vi "CLC_GEN3_L2_InPhaseCal_mW_BaseOnly.vi"() -> ()   [LabVIEW 2023, in "Clover_Cell.lvlib"]
uses:
  Clover_Cell.lvlib
  lib/Anritsu Signal Analyzer Series/Anritsu Signal Analyzer Series.lvlib
  lib/ELTA/ELTA.lvlib
panel:
  in  "Base_Gain":i32
  in  "Base_Phase":i32
  in  "Base_Ch":i32
  in  "Daul_Ch_Phase_Sweep":bool
  in  "SweepSwitch?":u16(ring) items=["NoSweep(Single)", "Sweep"]
  in  "SweepMode":u16(ring) items=["Phase", "Gain"]
  in  "Method":u16(ring)=1 items=["dBm"=1, "mW"=2]
  in  "Polarity":u16(ring) items=["H", "V"]
  in  "VISA resource name":refnum<visa-resource-name>="TCPIP0::192.168.100.230::inst0::INSTR"
  in  "CenterFreq(GHz)":dbl=28.0
  in  "AvgTimes":i32=3
  in  "Single_Ch_Phase_Sweep":bool
  in  "TRXmode":u16(ring)=1 items=["Rx"=2, "Tx"=1]
  out "GainStep":i32=63
  out "PhaseStep":i32=63
  out "Channel":i32=63
  out "Total mW":dbl format="%.7f"
  out "Total dBm":dbl format="%.7f"
  out "Ref. mW":dbl format="%.7f"
  out "Ref. dBm":dbl format="%.7f"
  out "Main mW":dbl format="%.7f"
  out "Main dBm":dbl format="%.7f"
  out "Data":dbl[][](array[numeric])
  out "FileNAME_Single":string
  out "Spectrum Analyzer":dbl[](graph)
  out "CurrentData":dbl[](array[numeric])
  out "Duration":dbl
  out "TotalTime":dbl format="%.2f"
  out "StopTime":timestamp=timestamp(3663835912.033212 s since 1904-01-01)
  out "FileNAME_Dual":string
  out "StartTime":timestamp=timestamp(3663835741.875155 s since 1904-01-01)
  out "TX/RX":u16=1
  out "error out":errorcluster
  out "output cluster":T1={"address"="192.168.100.111", "remote port or service name"=5025, "timeout ms (60000)"=10000}
  out "Operating \nChannel(s)":bool[][](array[boolean])
  out "OK?":bool
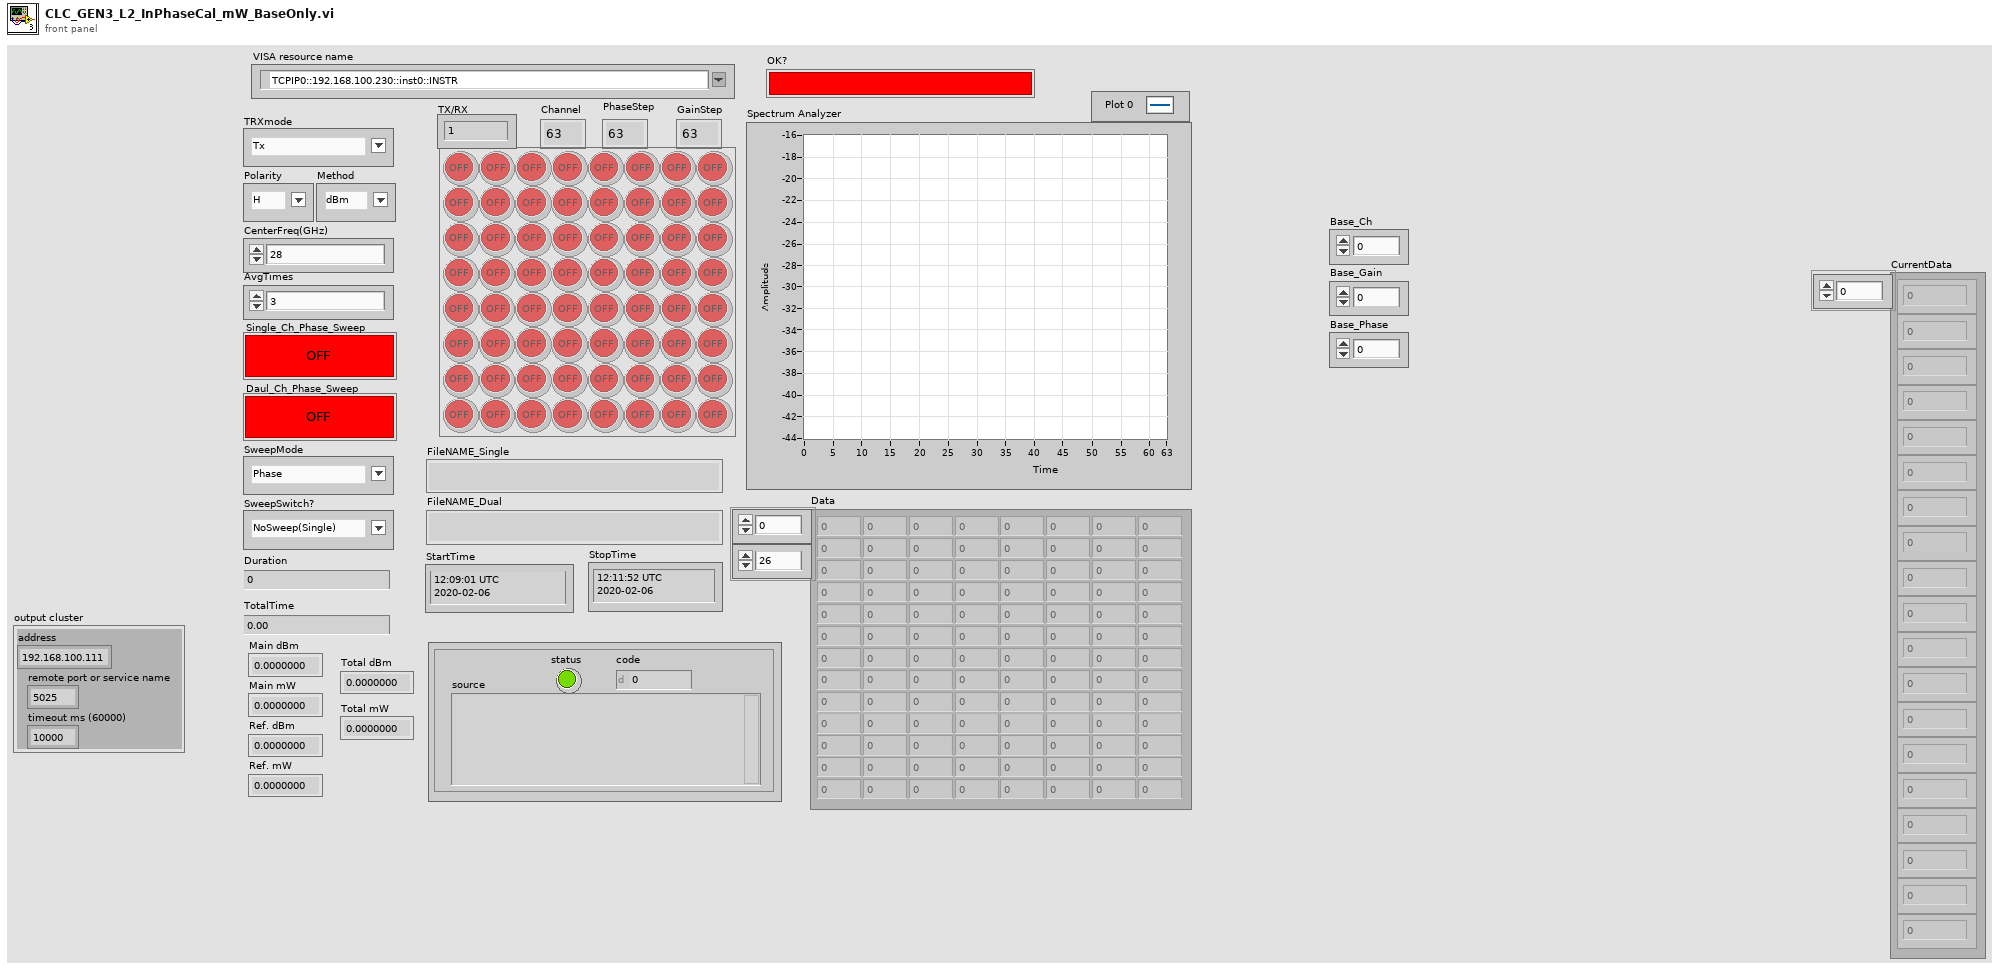
[diagram p1: front panel]
types:
  T1 = cluster{"address":string, "remote port or service name":u16, "timeout ms (60000)":i32}
  T2 = cluster{"Mode":u16, "Polarity":u16, "CH_ON/OFF":u16, "Channel":i32, "Gain":i32, "Phase":i32}
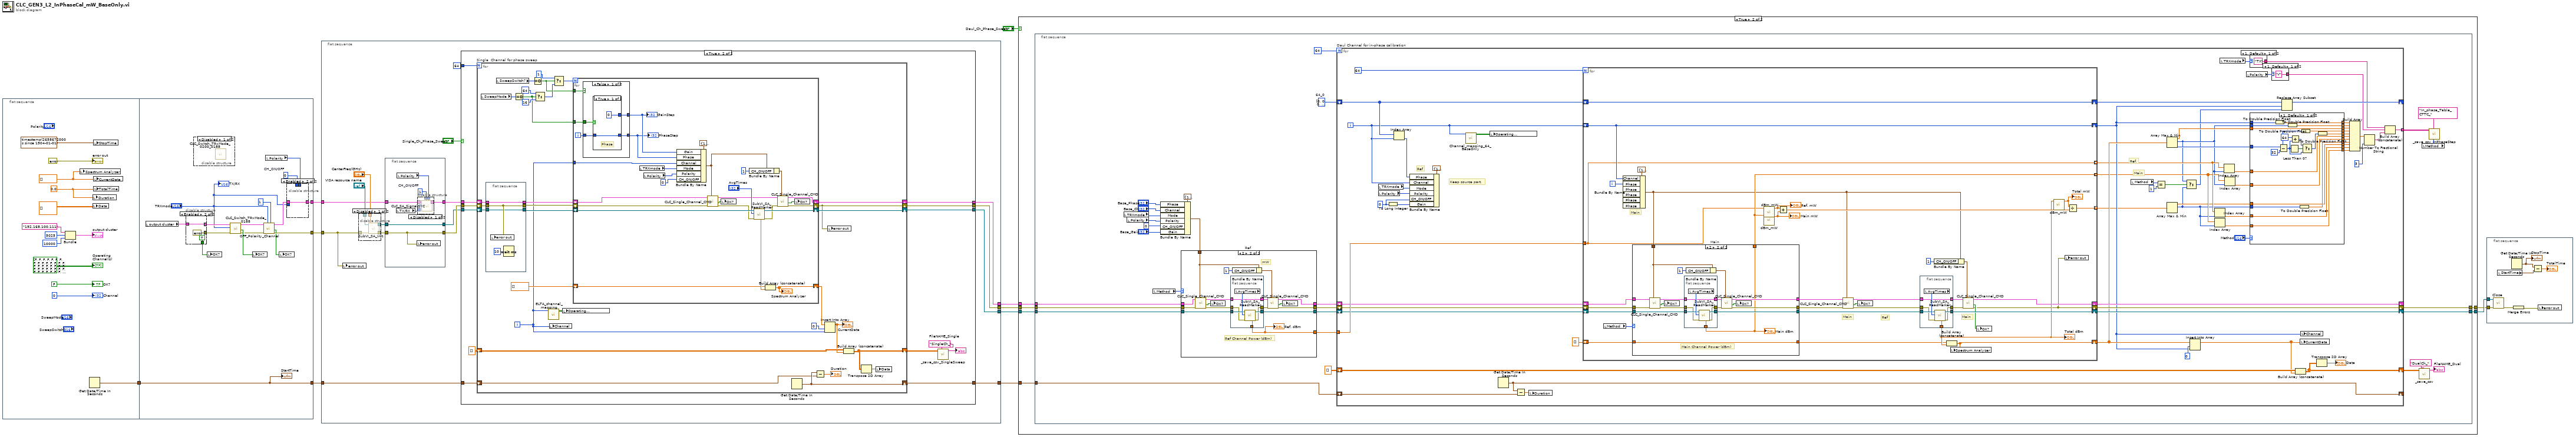
[diagram p0: block diagram]
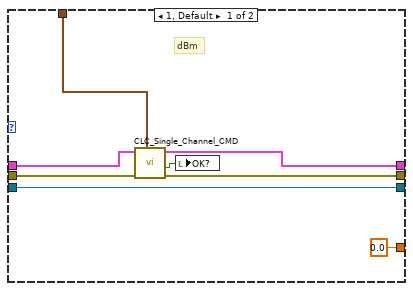
[diagram p3: hidden frame]
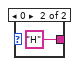
[diagram p4: hidden frame]
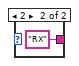
[diagram p5: hidden frame]
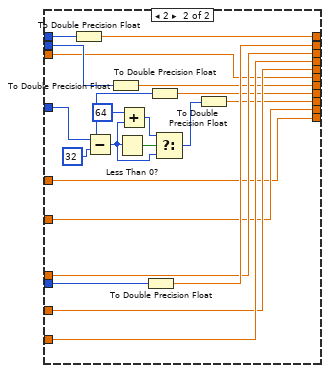
[diagram p6: hidden frame]
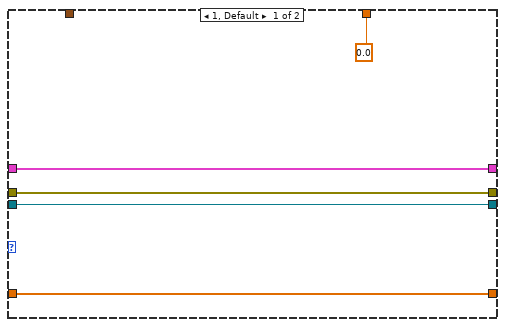
[diagram p7: hidden frame]
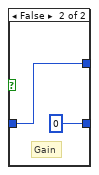
[diagram p10: hidden frame]
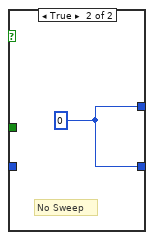
[diagram p11: hidden frame]
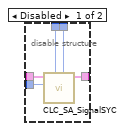
[diagram p14: hidden frame]
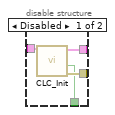
[diagram p15: hidden frame]
diagram:
  n1 = flat-sequence {
    tunnel: [w12] -> w11
    tunnel: w11 -> [w28]
    tunnel: [w31] -> w2
    tunnel: [w35] -> w3
    tunnel: [w28] -> w10
    frame #0 {
      w16 = dbl[] []
      w19 = 0.0 ("TotalTime")
      n2 = Bundle("address"="192.168.100.111", "remote port or service name"=u16 5025, "timeout ms (60000)"=10000) -> (→"output cluster":T1)  [unwired: 1 in]
      n3 = local write "Spectrum Analyzer"(w16) -> ()
      n4 = Get Date/Time In Seconds() -> (seconds since 1Jan1904=w12:timestamp)
      n5 = local write "Duration"(w19) -> ()
      n6 = local write "Data"(dbl[][] []) -> ()
      n7 = local write "StopTime"(timestamp(2658672000.001 s since 1904-01-01) ("StopTime")) -> ()
      n8 = local write "CurrentData"(w16) -> ()
      n9 = local write "TotalTime"(w19) -> ()
      "error out" <- errorcluster {"status"=FALSE, "code"=0, "source"=""} ("error out")
      "Operating \nChannel(s)" <- bool[][] [[FALSE, FALSE, FALSE, FALSE, FALSE, FALSE, FALSE, FALSE], [FALSE, FALSE, FALSE, FALSE, FALSE, FALSE, FALSE, FALSE], [FALSE, FALSE, FALSE, FALSE, FALSE, FALSE, FALSE, FALSE], [FALSE, FALSE, FALSE, FALSE, FALSE, FALSE, FALSE, FALSE], [FALSE, FALSE, FALSE, FALSE, FALSE, FALSE, FALSE, FALSE], [FALSE, FALSE, FALSE, FALSE, FALSE, FALSE, FALSE, FALSE], [FALSE, FALSE, FALSE, FALSE, FALSE, FALSE, FALSE, FALSE], [FALSE, FALSE, FALSE, FALSE, FALSE, FALSE, FALSE, FALSE]] ("Operating \nChannel(s)")
      "Channel" <- 0 ("Channel")
      "OK?" <- FALSE ("OK?")
    }
    frame #1 {
      w30 = u16 0  # CH_ON/OFF
      n10 = local read "output cluster"() -> (w40:T1)
      n11 = disable-structure shown="Enabled" {
        disable-tunnel: w40 -> [w50 w53]
        disable-tunnel: [w49 w53] -> w39
        disable-tunnel: [w48 errorcluster {"status"=FALSE, "code"=0, "source"=""} ("error in (no error)")] -> w37
        disable-tunnel: [w47 TRUE ("OK?")] -> w29
        frame Disabled {
          n12 = call "CLC_Init.vi"("TCPIPin"=w50) -> ("error out"=w48:errorcluster, "Status"=w47:bool, "TCPIPin 2"=w49:T1)  [unwired: 8 in]
        }
        frame Enabled {
        }
      }
      n13 = disable-structure shown="Disabled" {
        frame Disabled {
          n14 = call "CLC_Switch_TRxMode_0200_0188.vi"() -> ()  [unwired: 9 in, 3 out]
        }
        frame Enabled {
        }
      }
      n15 = local write "OK?"(w29) -> ()
      n16 = call "CLC_Switch_TRxMode_0188.vi"("error in (no error)"=w37, "Text Ring"="TRXmode", "TCPIPin"=w39) -> ("error out"=w36:errorcluster, "OK?"=w38:bool, "TCPIPin 2"=w34:T1)  [unwired: 6 in]
      n17 = local write "OK?"(w38) -> ()
      n18 = call "OFF_Polarity_Channel.vi"("CH_ON:0/OFF:1"=u16 1, "Mode"="TRXmode", "error in"=w36, "TCPIPin"=w34) -> ("error out"=w35:errorcluster, "OK?"=w33:bool, "TCPIPout"=w32:T1)  [unwired: 5 in]
      n19 = local read "Polarity"() -> (w26:u16)
      n20 = local write "OK?"(w33) -> ()
      n21 = disable-structure shown="Enabled" {
        disable-tunnel: w32 -> [w45 w46]
        disable-tunnel: [w44 w46] -> w31
        disable-tunnel: w30 -> [w43 _]
        disable-tunnel: w26 -> [w42 _]
        disable-tunnel: "TRXmode" -> [w41 _]
        frame Disabled {
          n22 = call "CLC_SA_SignalSYC.vi"("Polarity"=w42, "CH_ON/OFF"=w43, "Mode"=w41, "TCPIPin"=w45) -> ("TCPIPout"=w44:T1)  [unwired: 7 in]
        }
        frame Enabled {
        }
      }
      "StartTime" <- w28
      "TX/RX" <- "TRXmode"
    }
  }
  n23 = flat-sequence {
    tunnel: w10 -> [w67]
    tunnel: [w66] -> w9
    tunnel: [w65] -> w8
    tunnel: [w64] -> w7
    tunnel: [w63] -> w4
    tunnel: w3 -> [w61]
    tunnel: w2 -> [w58]
    frame #0 {
      n24 = local write "error out"(w61) -> ()
      n25 = disable-structure shown="Disabled" {
        disable-tunnel: "VISA resource name" -> [w74 w75]
        disable-tunnel: [w73 w76] -> w62
        disable-tunnel: w61 -> [w72 w76]
        disable-tunnel: "CenterFreq(GHz)" -> [w71 _]
        disable-tunnel: [w70 w75] -> w57
        frame Disabled {
          n26 = call "SubVI_SA_Init.vi"("error in (no error)"=w72, "CenterFreq(GHz) 2"=w71, "VISA resource name"=w74) -> ("error out 2"=w73:errorcluster, "VISA resource name out"=w70:refnum<visa-resource-name>)  [unwired: 6 in, 1 out]
        }
        frame Enabled {
        }
      }
      n27 = flat-sequence {
        tunnel: w62 -> [w171]
        tunnel: [w171] -> w59
        tunnel: w58 -> [w169]
        tunnel: w57 -> [w170]
        tunnel: [w170] -> w56
        tunnel: [w168] -> w55
        frame #0 {
          w167 = u16 1  # CH_ON/OFF
          n28 = local read "TX/RX"() -> (w165:u16)
          n29 = local read "Polarity"() -> (w166:u16)
          n30 = local write "error out"(w171) -> ()
          n31 = disable-structure shown="Disabled" {
            disable-tunnel: w169 -> [w176 w177]
            disable-tunnel: [w175 w177] -> w168
            disable-tunnel: w167 -> [w174 _]
            disable-tunnel: w166 -> [w173 _]
            disable-tunnel: w165 -> [w172 _]
            frame Disabled {
              n32 = call "CLC_SA_SignalSYC.vi"("Polarity"=w173, "CH_ON/OFF"=w174, "Mode"=w172, "TCPIPin"=w176) -> ("TCPIPout"=w175:T1)  [unwired: 7 in]
            }
            frame Enabled {
            }
          }
        }
      }
      n33 = case shown="True" "Single_Ch_Phase_Sweep" {
        tunnel: 64 -> [_ w93]
        tunnel: w67 -> [w77 w92]
        tunnel: [w78 w91] -> w66
        tunnel: [w79 w90] -> w65
        tunnel: [w80 w89] -> w64
        tunnel: [w77 w88] -> w63
        tunnel: w59 -> [w79 w87]
        tunnel: w56 -> [w78 w86]
        tunnel: w55 -> [w80 w85]
        frame False {
        }
        frame True {
          n34 = for "Single  Channel for phase sweep" {
            N: w93 -> [_]
            shift-right: [w123] -> w89
            shift-left: w85 -> [w109]
            shift-right: [w118] -> w90
            shift-left: w87 -> [w111]
            shift-right: [w122] -> w91
            shift-left: w86 -> [w108]
            shift-right: [w116] -> w82
            shift-left: dbl[][] [] -> [w117]
            shift-right: [w120] -> w88
            shift-left: w92 -> [w119]
            i -> [w94]
            n35 = local read "SweepMode"() -> (w103:u16)
            n36 = flat-sequence {
              tunnel: [w125] -> w107
              tunnel: w111 -> [w126]
              tunnel: [w126] -> w110
              tunnel: w109 -> [w125]
              tunnel: w108 -> [w124]
              tunnel: [w124] -> w106
              frame #0 {
                n37 = local write "error out"(w126) -> ()
                n38 = Wait (ms)(milliseconds to wait=u32 10) -> ()  [unwired: 1 out]
              }
            }
            n39 = local read "SweepSwitch?"() -> (w102:u16)
            n40 = Equal To 0?(x=w103) -> (x = 0?=w95:bool)
            n41 = Equal To 0?(x=w102) -> (x = 0?=w96:bool)
            n42 = Select(t=64, s=w95, f=16) -> (s? t:f=w97:i32)
            n43 = call "ELTA_channel_mapping.vi"("Ch_1_ref"=w94) -> ("Operating \nChannel(s)"=w104:bool[][])  [unwired: 10 in]
            n44 = local write "Channel"(w94) -> ()
            n45 = Select(t=1, s=w96, f=w97) -> (s? t:f=w100:i32)
            n46 = local write "Operating \nChannel(s)"(w104) -> ()
            n47 = for {
              N: w100 -> [_]
              shift-right: [w137] -> w123
              shift-left: w107 -> [w147]
              shift-right: [w139] -> w118
              shift-left: w110 -> [w149]
              shift-right: [w154] -> w122
              shift-left: w106 -> [w155]
              shift-right: [w150] -> w115
              shift-left: dbl[] [] -> [w151]
              tunnel: w94 -> [w144]
              tunnel: w96 -> [w132]
              tunnel: w95 -> [w129]
              i -> [w128]
              n48 = case shown="False" w132 {
                tunnel: [w156 w164] -> w131
                tunnel: [w157 w164] -> w130
                tunnel: w129 -> [w159 _]
                tunnel: w128 -> [w158 _]
                frame False {
                  n49 = case shown="True" w159 {
                    tunnel: w158 -> [w161 w162]
                    tunnel: [w161 0] -> w157
                    tunnel: [0 w162] -> w156
                    frame True {
                      # "Phase"
                    }
                    frame False {
                      # "Gain"
                    }
                  }
                }
                frame True {
                  w164 = 0
                  # "No Sweep"
                }
              }
              "PhaseStep" <- w130
              "GainStep" <- w131
              n50 = local read "TRXmode"() -> (w143:u16)
              n51 = local read "Polarity"() -> (w142:u16)
              n52 = Bundle By Name(cluster=T2 {"Mode"=1, "Polarity"=1, "CH_ON/OFF"=1, "Channel"=0, "Gain"=0, "Phase"=0} ("Channel params"), "Gain"=w131, "Phase"=w130, "Channel"=w144, "Mode"=w143, "Polarity"=w142, "CH_ON/OFF"=u16 0) -> (w136:T2)
              n53 = call "CLC_Single_Channel_CMD.vi"("Channel params"=w136, "error in"=w149, "TCPIPin"=w147) -> ("error out"=w148:errorcluster, "OK?"=w145:bool, "TCPIPout"=w138:T1)  [unwired: 6 in]
              n54 = local write "OK?"(w145) -> ()
              n55 = Bundle By Name(cluster=w136, "CH_ON/OFF"=u16 1) -> (w134:T2)
              n56 = call "SubVI_SA_ReadMarker.vi"("error in (no error)"=w148, "AvgTimes"="AvgTimes", "VISA resource name"=w155) -> ("error out"=w140:errorcluster, "VISA resource name out"=w154:refnum<visa-resource-name>, "Marker Power"=w152:dbl)  [unwired: 5 in, 1 out]
              n57 = Build Array (concatenate)(w151, w152) -> (w150:dbl[])
              "Spectrum Analyzer" <- w150
              n58 = call "CLC_Single_Channel_CMD.vi"("Channel params"=w134, "error in"=w140, "TCPIPin"=w138) -> ("error out"=w139:errorcluster, "OK?"=w133:bool, "TCPIPout"=w137:T1)  [unwired: 6 in]
              n59 = local write "OK?"(w133) -> ()
            }
            n60 = Get Date/Time In Seconds() -> (seconds since 1Jan1904=w120:timestamp)
            n61 = Subtract(x=w120, y=w119) -> (x-y=→"Duration":dbl)
            n62 = Insert Into Array(array=w115, index=0, new element=w94) -> (w113:dbl[])
            "CurrentData" <- w113
            n63 = local write "error out"(w118) -> ()
            n64 = Build Array (concatenate)(w117, w113) -> (w116:dbl[][])
            n65 = Transpose 2D Array(2D array=w116) -> (transposed array=w105:dbl[][])
            n66 = local write "Data"(w105) -> ()
          }
          n67 = call "_save_csv_SingleSweep.vi"("delimiter (\\t)"="SingleCh_" ("delimiter (\\t)"), "Data"=w82) -> ("FileName"=→"FileNAME_Single":string)  [unwired: 9 in]
        }
      }
    }
  }
  n68 = case shown="True" "Daul_Ch_Phase_Sweep" {
    tunnel: w9 -> [w179 w185]
    tunnel: w8 -> [w178 w184]
    tunnel: w7 -> [_ w183]
    tunnel: [w179 w182] -> w6
    tunnel: [w178 w181] -> w5
    tunnel: w4 -> [_ w180]
    frame False {
    }
    frame True {
      n69 = flat-sequence {
        tunnel: w185 -> [w198]
        tunnel: w184 -> [w194]
        tunnel: w183 -> [w195]
        tunnel: [w212] -> w182
        tunnel: [w211] -> w181
        tunnel: w180 -> [w210]
        frame #0 {
          w208 = i32[] [0, 0, 0, 0, 0, 0, 0, 0, 0, 0, 0, 0, 0, 0, 0, 0, 0, 0, 0, 0, 0, 0, 0, 0, 0, 0, 0, 0, 0, 0, 0, 0, 0, 0, 0, 0, 0, 0, 0, 0, 0, 0, 0, 0, 0, 0, 0, 0, 0, 0, 0, 0, 0, 0, 0, 0, 0, 0, 0, 0, 0, 0, 0, 0]  # 64_0
          n70 = local read "TRXmode"() -> (w191:u16)
          n71 = local read "Polarity"() -> (w192:u16)
          n72 = local read "Method"() -> (w201:u16)
          n73 = Bundle By Name(cluster=T2 {"Mode"=1, "Polarity"=1, "CH_ON/OFF"=1, "Channel"=0, "Gain"=0, "Phase"=0} ("Channel params"), "Phase"="Base_Phase", "Channel"="Base_Ch", "Mode"=w191, "Polarity"=w192, "CH_ON/OFF"=u16 0, "Gain"="Base_Gain") -> (w189:T2)
          n74 = case "Ref" shown="2" w201 {
            tunnel: w194 -> [w216 w229]
            tunnel: [w219 w228] -> w197
            tunnel: w198 -> [w221 w227]
            tunnel: [w221 w226] -> w199
            tunnel: w195 -> [w217 w225]
            tunnel: [w218 w224] -> w196
            tunnel: [0.0 ("Marker Response") w223] -> w200
            tunnel: w189 -> [w215 w222]
            frame 1, Default {
              # "dBm"
              n75 = call "CLC_Single_Channel_CMD.vi"("Channel params"=w215, "error in"=w216, "TCPIPin"=w217) -> ("error out"=w219:errorcluster, "OK?"=w214:bool, "TCPIPout"=w218:T1)  [unwired: 6 in]
              n76 = local write "OK?"(w214) -> ()
            }
            frame 2 {
              # "mW"
              # "Ref Channel Power (dBm)"
              n77 = call "CLC_Single_Channel_CMD.vi"("Channel params"=w222, "error in"=w229, "TCPIPin"=w225) -> ("error out"=w236:errorcluster, "OK?"=w237:bool, "TCPIPout"=w235:T1)  [unwired: 6 in]
              n78 = local write "OK?"(w237) -> ()
              n79 = flat-sequence {
                tunnel: [w244] -> w226
                tunnel: [w242] -> w223
                tunnel: w227 -> [w241]
                tunnel: w236 -> [w240]
                tunnel: [w239] -> w231
                tunnel: w235 -> [w239]
                tunnel: [w238] -> w232
                frame #0 {
                  n80 = local read "AvgTimes"() -> (w243:i32)
                  n81 = call "SubVI_SA_ReadMarker.vi"("error in (no error)"=w240, "AvgTimes"=w243, "VISA resource name"=w241) -> ("error out"=w238:errorcluster, "VISA resource name out"=w244:refnum<visa-resource-name>, "Marker Power"=w242:dbl)  [unwired: 5 in, 1 out]
                }
              }
              n82 = Bundle By Name(cluster=w222, "CH_ON/OFF"=u16 1) -> (w233:T2)
              n83 = call "CLC_Single_Channel_CMD.vi"("Channel params"=w233, "error in"=w232, "TCPIPin"=w231) -> ("error out"=w228:errorcluster, "OK?"=w234:bool, "TCPIPout"=w224:T1)  [unwired: 6 in]
              n84 = local write "OK?"(w234) -> ()
              "Ref. dBm" <- w223
            }
          }
          n85 = for "Daul Channel for in-phase calibration" {
            N: 64 -> [_]
            shift-right: [w310] -> _
            shift-left: w196 -> [w248]
            shift-right: [w307] -> w211
            shift-left: w197 -> [w247]
            shift-right: [w308] -> w212
            shift-left: w199 -> [w246]
            shift-right: [w302] -> w203
            shift-left: dbl[][] [] -> [w303]
            shift-right: [w306] -> _
            shift-left: w210 -> [w305]
            shift-right: [w296] -> _
            shift-left: w208 -> [w278]
            tunnel: [w250] -> w204 mode=indexing
            tunnel: w200 -> [w249]
            i -> [w245]
            w280 = u16 0 ("CH_ON/OFF")
            # "Keep source part,"
            # "Main"
            # "Ref."
            # "Ref"
            n86 = local read "TRXmode"() -> (w282:u16)
            n87 = local read "Polarity"() -> (w281:u16)
            n88 = To Long Integer(number=w280) -> (32bit integer=w279:i32)
            n89 = Index Array(array=w278, index=w245) -> (element=w277:i32)
            n90 = Bundle By Name(cluster=T2 {"Mode"=1, "Polarity"=1, "CH_ON/OFF"=1, "Channel"=0, "Gain"=0, "Phase"=0} ("Channel params"), "Phase"=w277, "Channel"=w245, "Mode"=w282, "Polarity"=w281, "CH_ON/OFF"=w280, "Gain"=w279) -> ()  [unwired: 1 out]
            n91 = call "Channel_mapping_64_BaseOnly.vi"("Channel IN"=w245) -> ("Operating \nChannel(s)"=w284:bool[][])  [unwired: 10 in]
            n92 = local write "Operating \nChannel(s)"(w284) -> ()
            n93 = Get Date/Time In Seconds() -> (seconds since 1Jan1904=w306:timestamp)
            n94 = Subtract(x=w306, y=w305) -> (x-y=w304:dbl)
            n95 = local write "Duration"(w304) -> ()
            n96 = for {
              N: 64 -> [_]
              shift-right: [w359] -> w310
              shift-left: w248 -> [w369]
              shift-right: [w358] -> w307
              shift-left: w247 -> [w382]
              shift-right: [w390] -> w308
              shift-left: w246 -> [w381]
              shift-right: [w384] -> w297
              shift-left: dbl[] [] -> [w371]
              shift-right: [w388] -> w295
              shift-left: w278 -> [w388]
              shift-right: [w365] -> w294
              shift-left: w245 -> [w365]
              tunnel: [w362] -> w287 mode=indexing
              tunnel: [w375] -> w286 mode=indexing
              tunnel: [w376] -> w293 mode=indexing
              tunnel: w249 -> [w362]
              i -> [w366]
              # "Main"
              # "Main"
              # "Ref"
              # "Main"
              n97 = local read "Method"() -> (w372:u16)
              n98 = Bundle By Name(cluster=T2 {"Mode"=1, "Polarity"=1, "CH_ON/OFF"=1, "Channel"=0, "Gain"=0, "Phase"=0} ("Channel params"), "Channel"=w365, "Phase"=w366) -> (w364:T2)  [unwired: 4 in]
              n99 = case "Main" shown="2" w372 {
                tunnel: w382 -> [w393 w399]
                tunnel: w369 -> [w394 w400]
                tunnel: w381 -> [w392 w398]
                tunnel: [w394 w404] -> w380
                tunnel: [w393 w403] -> w379
                tunnel: [w392 w402] -> w378
                tunnel: w364 -> [_ w401]
                tunnel: [0.0 ("Marker Response") w396] -> w375
                tunnel: w371 -> [w391 w397]
                tunnel: [w391 w397] -> w370
                frame 1, Default {
                }
                frame 2 {
                  # "Main Channel Power (dBm)"
                  n100 = call "CLC_Single_Channel_CMD.vi"("Channel params"=w401, "error in"=w399, "TCPIPin"=w400) -> ("error out"=w406:errorcluster, "OK?"=w405:bool, "TCPIPout"=w407:T1)  [unwired: 6 in]
                  n101 = local write "OK?"(w405) -> ()
                  n102 = flat-sequence {
                    tunnel: [w419] -> w402
                    tunnel: [w417] -> w396
                    tunnel: w398 -> [w416]
                    tunnel: w406 -> [w415]
                    tunnel: [w414] -> w412
                    tunnel: w407 -> [w414]
                    tunnel: [w413] -> w411
                    frame #0 {
                      n103 = local read "AvgTimes"() -> (w418:i32)
                      n104 = call "SubVI_SA_ReadMarker.vi"("error in (no error)"=w415, "AvgTimes"=w418, "VISA resource name"=w416) -> ("error out"=w413:errorcluster, "VISA resource name out"=w419:refnum<visa-resource-name>, "Marker Power"=w417:dbl)  [unwired: 5 in, 1 out]
                    }
                  }
                  n105 = Bundle By Name(cluster=w401, "CH_ON/OFF"=u16 1) -> (w410:T2)
                  n106 = call "CLC_Single_Channel_CMD.vi"("Channel params"=w410, "error in"=w411, "TCPIPin"=w412) -> ("error out"=w403:errorcluster, "OK?"=w408:bool, "TCPIPout"=w404:T1)  [unwired: 6 in]
                  n107 = local write "OK?"(w408) -> ()
                  "Main dBm" <- w396
                }
              }
              n108 = call "dBm_mW.vi"("dBm"=w362) -> ("mW"=w368:dbl)  [unwired: 10 in]
              "Ref. mW" <- w368
              n109 = call "dBm_mW.vi"("dBm"=w375) -> ("mW"=w367:dbl)  [unwired: 10 in]
              "Main mW" <- w367
              n110 = Add(x=w368, y=w367) -> (x+y=w377:dbl)
              n111 = call "CLC_Single_Channel_CMD.vi"("Channel params"=w364, "error in"=w379, "TCPIPin"=w380) -> ("error out"=w360:errorcluster, "OK?"=w389:bool, "TCPIPout"=w361:T1)  [unwired: 6 in]
              n112 = local write "OK?"(w389) -> ()
              n113 = flat-sequence {
                tunnel: [w426] -> w390
                tunnel: [w424] -> w374
                tunnel: w378 -> [w423]
                tunnel: w360 -> [w422]
                tunnel: [w421] -> w387
                tunnel: w361 -> [w421]
                tunnel: [w420] -> w383
                frame #0 {
                  n114 = local read "AvgTimes"() -> (w425:i32)
                  n115 = call "SubVI_SA_ReadMarker.vi"("error in (no error)"=w422, "AvgTimes"=w425, "VISA resource name"=w423) -> ("error out"=w420:errorcluster, "VISA resource name out"=w426:refnum<visa-resource-name>, "Marker Power"=w424:dbl)  [unwired: 5 in, 1 out]
                }
              }
              n116 = Bundle By Name(cluster=w364, "CH_ON/OFF"=u16 1) -> (w385:T2)
              n117 = Build Array (concatenate)(w370, w374) -> (w384:dbl[])
              n118 = local write "Spectrum Analyzer"(w384) -> ()
              n119 = call "CLC_Single_Channel_CMD.vi"("Channel params"=w385, "error in"=w383, "TCPIPin"=w387) -> ("error out"=w358:errorcluster, "OK?"=w386:bool, "TCPIPout"=w359:T1)  [unwired: 6 in]
              n120 = local write "OK?"(w386) -> ()
              n121 = call "dBm_mW.vi"("dBm"=w374) -> ("mW"=w373:dbl)  [unwired: 10 in]
              "Total mW" <- w373
              n122 = local write "error out"(w358) -> ()
              n123 = Divide(x=w373, y=w377) -> (x/y=w376:dbl)
              "Total dBm" <- w374
            }
            n124 = local read "Method"() -> (w264:u16)
            n125 = Equal?(x=w264, y=u16 1) -> (x = y?=w262:bool)
            n126 = Array Max & Min(array=w297) -> (max value=w274:dbl, max index (indices)=w261:i32, min index (indices)=w285:i32)  [unwired: 1 out]
            n127 = Array Max & Min(array=w293) -> (max value=w268:dbl, max index (indices)=w260:i32)  [unwired: 2 out]
            n128 = Select(t=w261, s=w262, f=w260) -> (s? t:f=w259:i32)
            n129 = Insert Into Array(array=w297, index=0, new element=w294) -> (w298:dbl[])
            n130 = Index Array(array=w287, index=w260) -> (element=w267:dbl)
            n131 = Index Array(array=w286, index=w260) -> (element=w266:dbl)
            n132 = local read "TRXmode"() -> (w255:u16)
            n133 = Index Array(array=w287, index=w261) -> (element=w272:dbl)
            n134 = Index Array(array=w286, index=w261) -> (element=w271:dbl)
            n135 = local read "Polarity"() -> (w254:u16)
            n136 = case shown="1, Default" w255 {
              tunnel: ["TX" "RX"] -> w251
              frame 1, Default {
              }
              frame 2 {
              }
            }
            n137 = case shown="1, Default" "Method" {
              tunnel: w294 -> [w329 w350]
              tunnel: [w315 w344] -> w292
              tunnel: [w328 w343] -> w291
              tunnel: [w327 w342] -> w290
              tunnel: [w326 w346] -> w289
              tunnel: [w325 w339] -> w288
              tunnel: w285 -> [w324 w349]
              tunnel: w260 -> [w323 w348]
              tunnel: w261 -> [w322 w347]
              tunnel: w274 -> [w315 w341]
              tunnel: [w316 w345] -> w275
              tunnel: [w321 w341] -> w273
              tunnel: w272 -> [w321 w336]
              tunnel: w271 -> [w320 w337]
              tunnel: [w320 w340] -> w270
              tunnel: [w319 w338] -> w269
              tunnel: w268 -> [w319 w344]
              tunnel: w267 -> [w318 w342]
              tunnel: w266 -> [w317 w343]
              tunnel: [w317 w336] -> w265
              tunnel: [w318 w337] -> w258
              frame 1, Default {
                n138 = To Double Precision Float(number=w329) -> (double precision float=w326:dbl)
                n139 = Subtract(x=w324, y=32) -> (x-y=w331:i32)
                n140 = To Double Precision Float(number=w322) -> (double precision float=w316:dbl)
                n141 = Less Than 0?(x=w331) -> (x < 0?=w334:bool)
                n142 = Add(x=64, y=w331) -> (x+y=w332:i32)
                n143 = To Double Precision Float(number=w323) -> (double precision float=w325:dbl)
                n144 = To Double Precision Float(number=w324) -> (double precision float=w328:dbl)
                n145 = Select(t=w332, s=w334, f=w331) -> (s? t:f=w330:i32)
                n146 = To Double Precision Float(number=w330) -> (double precision float=w327:dbl)
              }
              frame 2 {
                n147 = To Double Precision Float(number=w350) -> (double precision float=w346:dbl)
                n148 = Subtract(x=w349, y=32) -> (x-y=w352:i32)
                n149 = To Double Precision Float(number=w347) -> (double precision float=w340:dbl)
                n150 = Less Than 0?(x=w352) -> (x < 0?=w355:bool)
                n151 = Add(x=64, y=w352) -> (x+y=w353:i32)
                n152 = To Double Precision Float(number=w348) -> (double precision float=w345:dbl)
                n153 = To Double Precision Float(number=w349) -> (double precision float=w339:dbl)
                n154 = Select(t=w353, s=w355, f=w352) -> (s? t:f=w351:i32)
                n155 = To Double Precision Float(number=w351) -> (double precision float=w338:dbl)
              }
            }
            n156 = case shown="1, Default" w254 {
              tunnel: ["V" "H"] -> w252
              frame 1, Default {
              }
              frame 0 {
              }
            }
            n157 = Replace Array Subset(array=w295, new element=w259, index=w294) -> (w296:i32[])
            n158 = Build Array (concatenate)(w303, w298) -> (w302:dbl[][])
            n159 = local write "CurrentData"(w298) -> ()
            n160 = local write "Channel"(w294) -> ()
            n161 = Transpose 2D Array(2D array=w302) -> (transposed array=→"Data":dbl[][])
            n162 = Build Array(w289, w275, w292, w291, w290, w273, w270, w288, w269, w258, w265) -> (w256:dbl[])
            n163 = Number To Fractional String(number=w256, precision (6)=i16 3) -> (F-format string=w253:string[])  [unwired: 2 in]
            n164 = Build Array (concatenate)(w251, w252, w253) -> (w250:string[])
          }
          n165 = call "_save_csv.vi"("delimiter (\\t)"="DualCh_" ("delimiter (\\t)"), "Data"=w203) -> ("FileName"=→"FileNAME_Dual":string)  [unwired: 9 in]
          n166 = local read "Method"() -> (w202:u16)
          n167 = call "_save_csv_InPhaseStep.vi"("Method"=w202, "delimiter (\\t)"="In_phase_Table_CTTC_" ("delimiter (\\t)"), "dataInput"=w204) -> ()  [unwired: 8 in, 1 out]
        }
      }
    }
  }
  n168 = flat-sequence {
    tunnel: w6 -> [w432]
    tunnel: w5 -> [w431]
    frame #0 {
      n169 = call "Close.vi"("error in (no error)"=w431, "VISA resource name"=w432) -> ("error out"=w433:errorcluster)  [unwired: 9 in]
      n170 = local read "StartTime"() -> (w427:timestamp)
      n171 = Get Date/Time In Seconds() -> (seconds since 1Jan1904=w428:timestamp)
      "StopTime" <- w428
      n172 = Merge Errors(w433) -> (w430:errorcluster)
      n173 = Subtract(x=w428, y=w427) -> (x-y=→"TotalTime":dbl)
      n174 = local write "error out"(w430) -> ()
    }
  }
